vi "SetArrayVisibleGraphCtrl.vi"(9 "on/off":bool, 10 "활성 플롯들":u32[](array[numeric]), 11 "ref graph in":refnum<vi>) -> (3 "ref graph out":refnum<vi>)   [LabVIEW 2018, in "Library-Ctrl.lvlib"]
uses:
  Library-Ctrl.lvlib
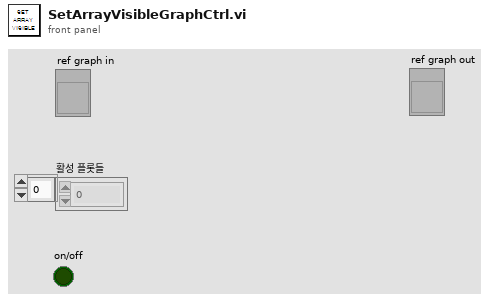
[diagram p1: front panel]
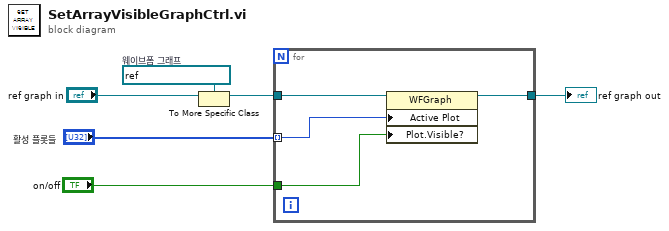
[diagram p0: block diagram]
diagram:
  w5 = refnum<vi> refnum  # 웨이브폼 그래프
  n1 = To More Specific Class(target class=w5, reference="ref graph in") -> (specific class reference=w4:refnum<vi>)  [unwired: 1 in, 1 out]
  n2 = for {
    tunnel: "on/off" -> [w8]
    tunnel: w4 -> [w10]
    tunnel: [w9] -> w3
    tunnel: "활성 플롯들" -> [w7] mode=indexing
    n3 = property class="WFGraph"(reference=w10, "Active Plot"=w7, "Plot.Visible?"=w8) -> (reference out=w9:refnum<vi>)  [unwired: 1 in, 1 out]
  }
  "ref graph out" <- w3
